vi "SR400 FlushBuffer.vi"(8 "error in (no error)":errorcluster, 11 "VISA Port In":refnum<visa-resource-name>="SR400") -> (0 "error out":errorcluster, 2 "data":string, 3 "VISA Port Out":refnum<visa-resource-name>="SR400")   [LabVIEW 2019]
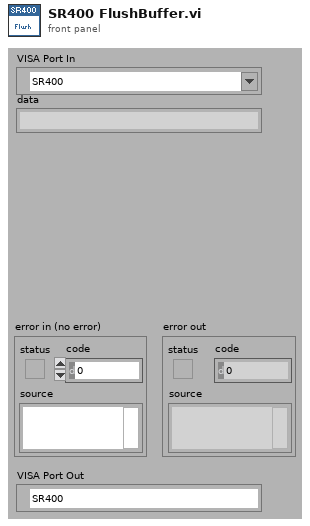
[diagram p1: front panel]
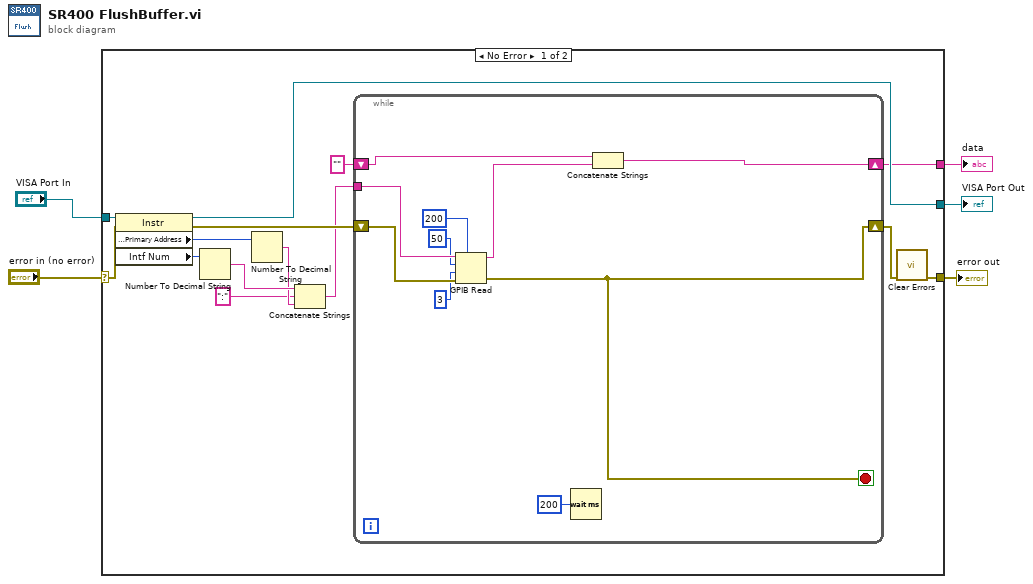
[diagram p0: block diagram]
diagram:
  n1 = case shown="No Error" "error in (no error)" {
    selector: "error in (no error)" -> [w19 w31]
    tunnel: [w8 w31] -> w4
    tunnel: "VISA Port In" -> [w18 w30]
    tunnel: [w9 w30] -> w2
    tunnel: [w7 _] -> w1
    frame No Error {
      n2 = property class="Instr"(reference=w18, error in=w19) -> (reference out=w9:refnum<visa-resource-name>, error out=w17:errorcluster, "GPIB Settings:Primary Address"=w16:u16, "Intf Num"=w14:u16)
      n3 = Number To Decimal String(number=w14) -> (decimal integer string=w13:string)  [unwired: 1 in]
      n4 = Number To Decimal String(number=w16) -> (decimal integer string=w12:string)  [unwired: 1 in]
      n5 = Concatenate Strings(w13, ":" ("string"), w12) -> (w10:string)
      n6 = while {
        tunnel: w10 -> [w28]
        shift-right: [w24] -> w15
        shift-left: w17 -> [w29]
        shift-right: [w21] -> w7
        shift-left: "" -> [w20]
        stop <- w24 stop-if-true
        n7 = GPIB Read(0:w28, 1:50 ("byte count"), 2:i16 3 ("mode (0)"), 3:w29, 4:200 ("timeout ms (488.2 global)")) -> (5:w22:string, 7:w24:errorcluster)  [unwired: 1 out]
        n8 = Wait (ms)(milliseconds to wait=u32 200) -> ()  [unwired: 1 out]
        n9 = Concatenate Strings(w20, w22) -> (w21:string)
      }
      n10 = call <vilib>:"Clear Errors.vi"("error in (no error)"=w15) -> ("error out"=w8:errorcluster)  [unwired: 5 in, 1 out]
    }
    frame Error {
    }
  }
  "error out" <- w4
  "VISA Port Out" <- w2
  "data" <- w1
